vi "GateCharge_Main.vi"() -> ()   [LabVIEW 2020]
uses:
  Global 1.vi
panel:
  in  "Median Filter Rank":i32=30
  out "Cluster 4":T1
  out "CURRENT RESULT":dbl[](array[numeric])
  in  "START TEST":bool
  out "Started":bool
  out "Elapsed time (minutes)":dbl
  out "start time":timestamp
  out "Oscilloscope Capture":waveform(dbl)[](graph)
  out "ALL RESULT Array":dbl[][](array[numeric])
  out "TEST#   |  Elapsed Time (minutes)":dbl[][](array[numeric])
  out "Gate Charge :\nTotal Test Time (minutes)":dbl
  in  "Finish?":bool
  out "Cluster 3":T2
  out "Cluster 2":T3
  out "Cluster 1":T4
  in  "Cluster : Setting":T5={"[-ve] VGE (V)"=0.0, "VCE (V)"=0.0, "ICE (A)"=0.0, "TEKTRONIX"="", "PROJECT #"="", "TEMPERATURE (C)"=0.0, "RG (Ohm)"=0.0, "DUT #"=1, "REQUEST #"="", "TEST #"=1, "IGE (mA)"=0.0, "[+ve] VGE (V)"=0.0}
  out "error out":errorcluster
  in  "error in (no error)":errorcluster
  # "PRODUCED BY : AFIQAH HASBULLAH ( SBN CZ ENG : 2022)"
  # "AC MODULE : GATE CHARGE"
  # "Column 0"
  # "Column 1"
  # "Column 2"
  # "Column 3"
  # "Column 4"
  # "Column 5"
  # "Column 6"
  # "Column 7"
  # "Column 8"
  # "Column 9"
  # "Column 10"
  # "Column 11"
  # "Column 12"
  # "Qge\n(nC)"
  # "Qgc\n(nC)"
  # "Qgtot\n(nC)"
  # "Vpl\n(V)"
  # "Vce"
  # "Ice"
  # "[-ve]Vge"
  # "[+ve]Vge"
  # "Rg"
  # "Temperature"
  # "DUT  #"
  # "TEST #"
  # "Ige"
  # "< Press 2 times >"
  # "Column 0"
  # "Column 1"
  # "Column 2"
  # "Column 3"
  # "Column 4"
  # "Column 5"
  # "Column 6"
  # "Column 7"
  # "Column 8"
  # "Column 9"
  # "Column 10"
  # "Column 11"
  # "Column 12"
  # "Qge\n(nC)"
  # "Qgc\n(nC)"
  # "Qgtot\n(nC)"
  # "Vpl\n(V)"
  # "Vce"
  # "Ice"
  # "[-ve]Vge"
  # "[+ve]Vge"
  # "Rg"
  # "Temperature"
  # "DUT  #"
  # "TEST #"
  # "Ige"
  # "Done  Qgtot  &  Vpl  Acquisition"
  # "Done  Qgc  Acquisition"
  # "Done  Qge  Acquisition"
  # "Done Exporting image of Overall Waveform"
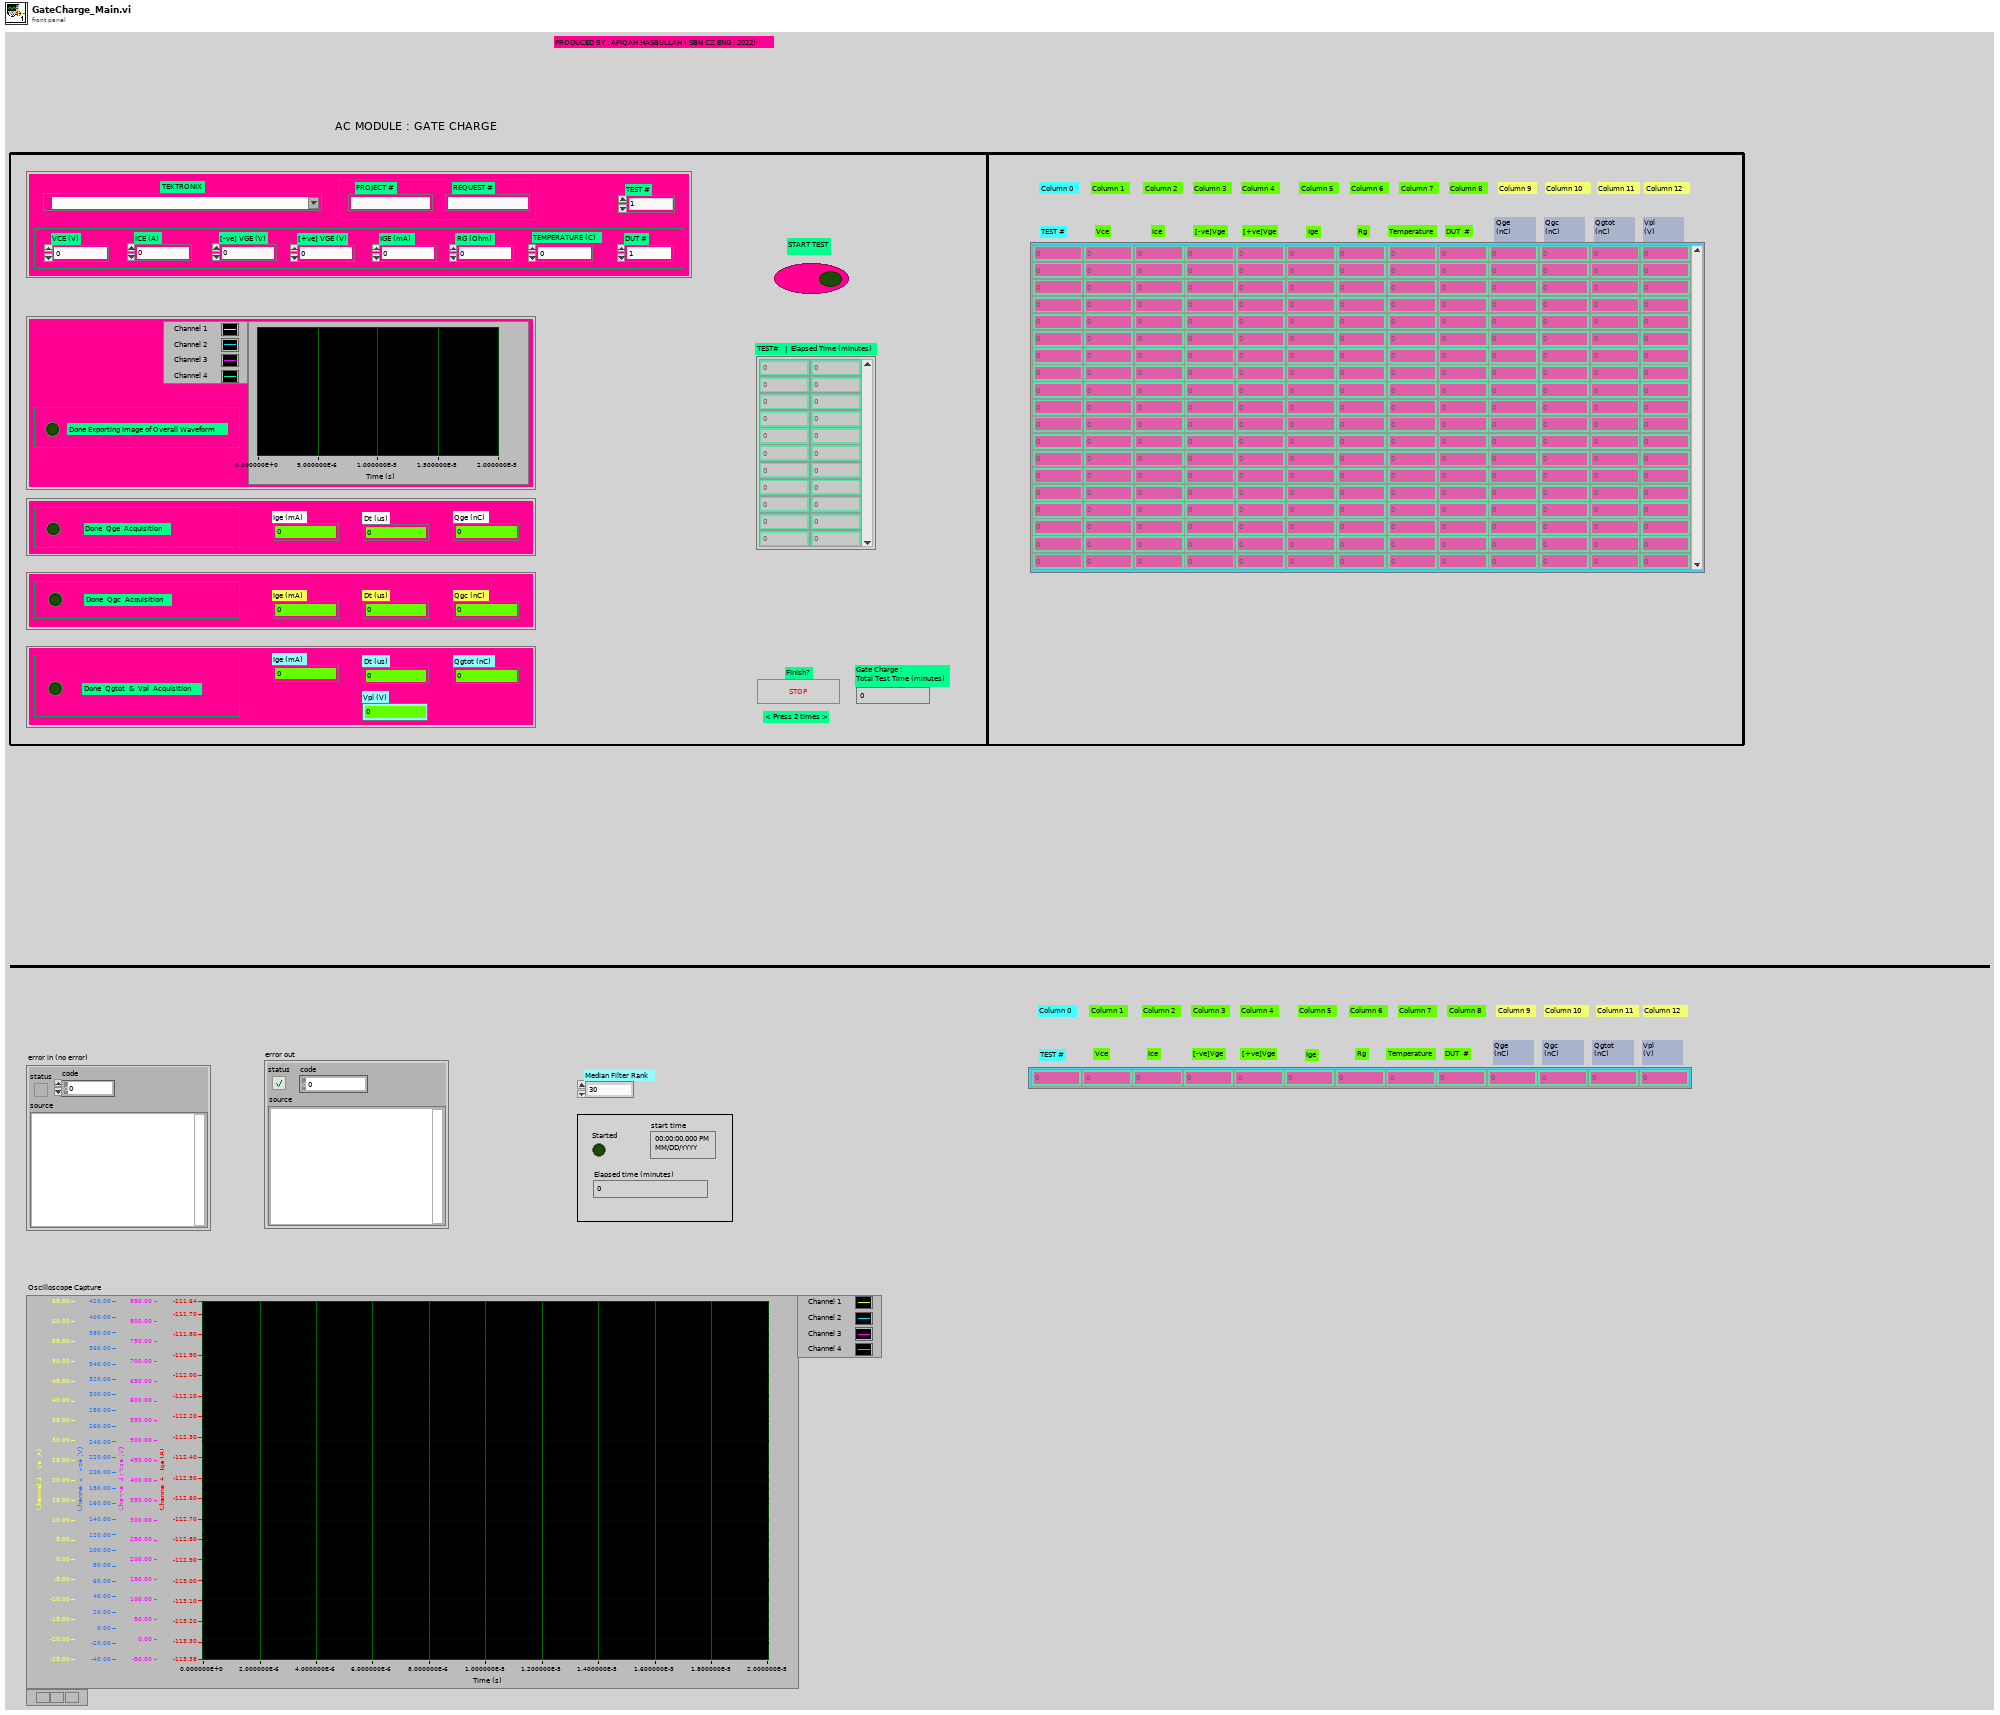
[diagram p1: front panel]
types:
  T1 = cluster{"Ige (mA)":dbl, "Qgtot (nC)":dbl, "Dt (us)":dbl, "LED 4":bool, "Vpl (V)":dbl}
  T2 = cluster{"Ige (mA)":dbl, "Dt (us)":dbl, "Qgc (nC)":dbl, "LED 3":bool}
  T3 = cluster{"Qge (nC)":dbl, "Ige (mA)":dbl, "Dt (us)":dbl, "LED 2":bool}
  T4 = cluster{"LED 1":bool, "Oscilloscope Capture":waveform(dbl)[]}
  T5 = cluster{"[-ve] VGE (V)":dbl, "VCE (V)":dbl, "ICE (A)":dbl, "TEKTRONIX":refnum<visa-resource-name>, "PROJECT #":string, "TEMPERATURE (C)":dbl, "RG (Ohm)":dbl, "DUT #":i32, "REQUEST #":string, "TEST #":i32, "IGE (mA)":dbl, "[+ve] VGE (V)":dbl}
  T6 = cluster{"Ige (mA)":dbl, "Qgtot (nC)":dbl, "Dt (us)":dbl, "LED 3":bool, "Vpl (V)":dbl}
  T7 = cluster{"Di/Dt (A/us)":dbl, "Di (A)":dbl, "Dt (ns)":dbl, "LED 2":bool}
  T8 = typedef "imagedata.ctl" = cluster{"image type":i32, "image depth":i32, "image":u8[], "mask":u8[], "colors":u32[], "Rectangle":cluster{"left":i16, "top":i16, "right":i16, "bottom":i16}}
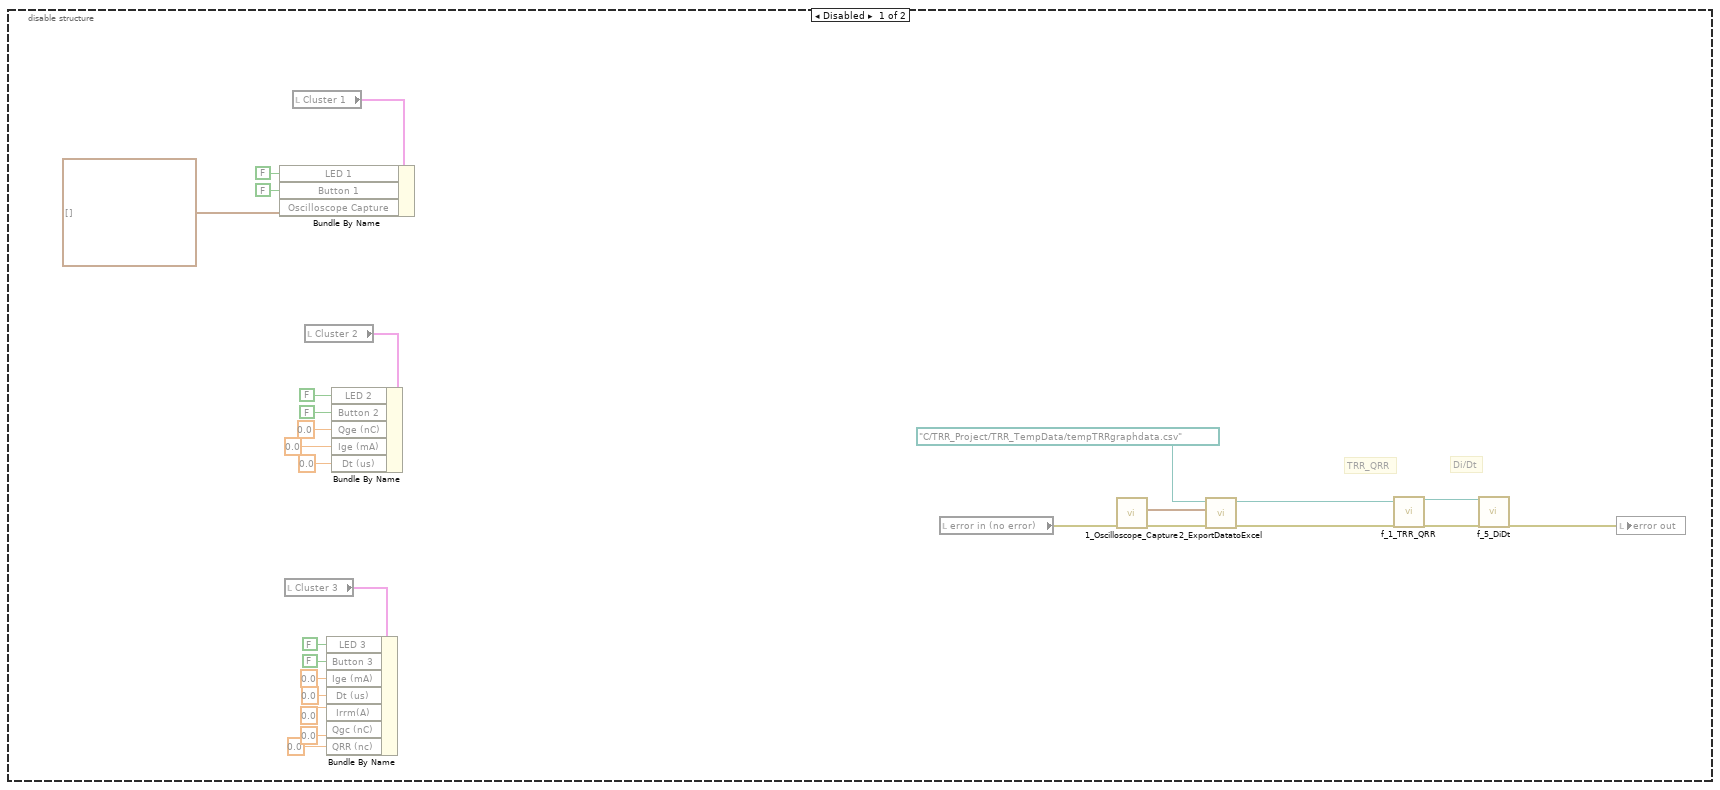
[diagram p3: hidden frame]
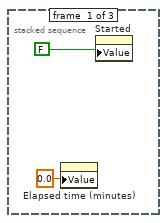
[diagram p4: hidden frame]
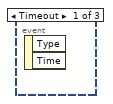
[diagram p6: hidden frame]
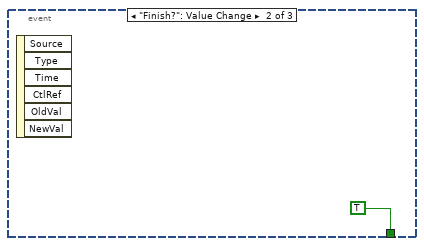
[diagram p7: hidden frame]
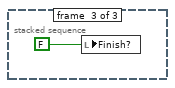
[diagram p9: hidden frame]
diagram:
  w1 = 30 ("Median Filter Rank")
  w18 = errorcluster {"status"=FALSE, "code"=0, "source"=""} ("error out")
  w5 = FALSE ("Started")
  w17 = 0.0 ("TRR :\nTotal Test Time (minutes)")
  n1 = flat-sequence {
    tunnel: [w28] -> w8
    tunnel: w8 -> [w29]
    tunnel: [w30] -> w7
    tunnel: w7 -> [w296]
    tunnel: [w291] -> w6
    tunnel: w6 -> [w322]
    frame #0 {
      # "IN"
      n2 = local read "error in (no error)"() -> (w28:errorcluster)
    }
    frame #1 {
      n3 = while {
        shift-right: [w33] -> w30
        shift-left: w29 -> [w32]
        stop <- w34 stop-if-true
        n4 = local read "START TEST"() -> (w36:bool)
        n5 = case shown="True" w36 {
          tunnel: w32 -> [w37 w57]
          tunnel: [w37 w38] -> w33
          frame False {
          }
          frame True {
            n6 = flat-sequence {
              tunnel: w57 -> [w59]
              tunnel: [w59] -> w51
              tunnel: w51 -> [w80]
              tunnel: [w80] -> w50
              tunnel: [w78] -> w49
              tunnel: [w77] -> w48
              tunnel: [w76] -> w47
              tunnel: [w75] -> w46
              tunnel: [w74] -> w45
              tunnel: [w73] -> w44
              tunnel: [w72] -> w43
              tunnel: [w70] -> w42
              tunnel: [w69] -> w41
              tunnel: w50 -> [w96]
              tunnel: [w96] -> w56
              tunnel: w49 -> [w95]
              tunnel: w48 -> [w94]
              tunnel: w47 -> [w93]
              tunnel: w46 -> [w92]
              tunnel: w45 -> [w91]
              tunnel: w44 -> [w90]
              tunnel: w43 -> [w89]
              tunnel: w42 -> [w82]
              tunnel: w41 -> [w81]
              tunnel: w56 -> [w123]
              tunnel: [w122] -> w55
              tunnel: w55 -> [w160]
              tunnel: [w156] -> w54
              tunnel: w54 -> [w198]
              tunnel: [w195] -> w40
              tunnel: w40 -> [w230]
              tunnel: [w228] -> w39
              tunnel: w39 -> [w269]
              tunnel: [w269] -> w53
              tunnel: w53 -> [w277]
              tunnel: [w277] -> w52
              tunnel: w52 -> [w286]
              tunnel: [w286] -> w38
              frame #0 {
                # "Initialize"
                n7 = local read "Median Filter Rank"() -> (w58:i32)
                n8 = Initialize Array(0.0 ("element"), 13 ("dimension size")) -> (w64:dbl[])
                n9 = local write "Cluster 4"(T6 {"Ige (mA)"=0.0, "Qgtot (nC)"=0.0, "Dt (us)"=0.0, "LED 3"=FALSE, "Vpl (V)"=0.0} ("Cluster 4")) -> ()
                n10 = local write "Cluster 3"(T2 {"Ige (mA)"=0.0, "Dt (us)"=0.0, "Qgc (nC)"=0.0, "LED 3"=FALSE} ("Cluster 3")) -> ()
                n11 = local write "Cluster 2"(T7 {"Di/Dt (A/us)"=0.0, "Di (A)"=0.0, "Dt (ns)"=0.0, "LED 2"=FALSE} ("Cluster 2")) -> ()
                n12 = local write "Oscilloscope Capture"(waveform(dbl)[] [] ("Oscilloscope Capture")) -> ()
                n13 = local write "CURRENT RESULT"(w64) -> ()
                n14 = Wait (ms)(milliseconds to wait=u32 500) -> ()  [unwired: 1 out]
                n15 = global write "Global 1.vi" "Median Filter Rank"(w58) -> ()
                n16 = local write "Cluster 1"(T4 {"LED 1"=FALSE, "Oscilloscope Capture"=[]} ("Cluster 1")) -> ()
              }
              frame #1 {
                n17 = local read "Cluster : Setting"() -> (w79:T5)
                n18 = Unbundle By Name(w79) -> ("TEST #"=w78:i32, "VCE (V)"=w77:dbl, "ICE (A)"=w76:dbl, "[-ve] VGE (V)"=w75:dbl, "[+ve] VGE (V)"=w74:dbl, "IGE (mA)"=w73:dbl, "RG (Ohm)"=w72:dbl, "TEMPERATURE (C)"=w70:dbl, "DUT #"=w69:i32)
                n19 = Wait (ms)(milliseconds to wait=u32 300) -> ()  [unwired: 1 out]
              }
              frame #2 {
                # "Column 8 = DUT#"
                # "Column 7 = Temperature"
                # "Column 6 = Rg"
                # "Column 5 = Ige"
                # "Column 4 = [+ve]Vge"
                # "Column 3 = [-ve]Vge"
                # "Column 2 = ICE"
                # "Column 1 = VCE"
                # "Column 0 = TEST#"
                # "Insert Test Condition"
                n20 = Wait (ms)(milliseconds to wait=u32 300) -> ()  [unwired: 1 out]
                n21 = local read "CURRENT RESULT"() -> (w87:dbl[])
                n22 = local read "CURRENT RESULT"() -> (w99:dbl[])
                n23 = local read "CURRENT RESULT"() -> (w101:dbl[])
                n24 = local read "CURRENT RESULT"() -> (w84:dbl[])
                n25 = local read "CURRENT RESULT"() -> (w103:dbl[])
                n26 = local read "CURRENT RESULT"() -> (w104:dbl[])
                n27 = local read "CURRENT RESULT"() -> (w111:dbl[])
                n28 = local read "CURRENT RESULT"() -> (w107:dbl[])
                n29 = local read "CURRENT RESULT"() -> (w109:dbl[])
                n30 = Replace Array Subset(array=w111, new element=w95, index=0) -> (w110:dbl[])
                n31 = Replace Array Subset(array=w109, new element=w94, index=1) -> (w108:dbl[])
                n32 = Replace Array Subset(array=w107, new element=w93, index=2) -> (w106:dbl[])
                n33 = Replace Array Subset(array=w104, new element=w92, index=3) -> (w105:dbl[])
                n34 = Replace Array Subset(array=w87, new element=w82, index=7) -> (w88:dbl[])
                n35 = Replace Array Subset(array=w99, new element=w89, index=6) -> (w98:dbl[])
                n36 = Replace Array Subset(array=w103, new element=w91, index=4) -> (w102:dbl[])
                n37 = Replace Array Subset(array=w101, new element=w90, index=5) -> (w100:dbl[])
                n38 = Replace Array Subset(array=w84, new element=w81, index=8) -> (w83:dbl[])
                n39 = local write "CURRENT RESULT"(w110) -> ()
                n40 = local write "CURRENT RESULT"(w108) -> ()
                n41 = local write "CURRENT RESULT"(w106) -> ()
                n42 = local write "CURRENT RESULT"(w105) -> ()
                n43 = local write "CURRENT RESULT"(w102) -> ()
                n44 = local write "CURRENT RESULT"(w100) -> ()
                n45 = local write "CURRENT RESULT"(w88) -> ()
                n46 = local write "CURRENT RESULT"(w98) -> ()
                n47 = local write "CURRENT RESULT"(w83) -> ()
              }
              frame #3 {
                n48 = Wait (ms)(milliseconds to wait=u32 300) -> ()  [unwired: 1 out]
                n49 = flat-sequence {
                  tunnel: w123 -> [w130]
                  tunnel: [w125] -> w120
                  tunnel: [w135] -> w119
                  tunnel: w120 -> [w134]
                  tunnel: [w151] -> w122
                  tunnel: w119 -> [w151]
                  frame #0 {
                    n50 = local read "Cluster : Setting"() -> (w129:T5)
                    n51 = Unbundle By Name(w129) -> ("TEKTRONIX"=w128:refnum<visa-resource-name>)
                    n52 = call "1_Oscilloscope_Capture.vi"("error in (no error)"=w130, "VISA Resource Name"=w128) -> ("error out"=w126:errorcluster, "Waveform Graph"=w124:waveform(dbl)[])  [unwired: 7 in, 1 out]
                    n53 = local write "Oscilloscope Capture"(w124) -> ()
                    n54 = local read "Cluster 1"() -> (w133:T4)
                    n55 = Bundle By Name(cluster=w133, "Oscilloscope Capture"=w124) -> (w132:T4)
                    n56 = local write "Cluster 1"(w132) -> ()
                    n57 = Wait (ms)(milliseconds to wait=u32 300) -> ()  [unwired: 1 out]
                    n58 = call "2_ExportDatatoExcel.vi"("error in (no error)"=w126, "Waveform Graph"=w124, "file path (IN)"=path "C:/GateCharge_Project/GateCharge_TempData/tempGateChargedata.csv") -> ("error out"=w125:errorcluster)  [unwired: 7 in, 1 out]
                  }
                  frame #1 {
                    w147 = "_"
                    n59 = local read "Cluster : Setting"() -> (w142:T5)
                    n60 = Unbundle By Name(w142) -> ("PROJECT #"=w139:string, "REQUEST #"=w138:string, "TEST #"=w141:i32)
                    n61 = invoke on="Oscilloscope Capture" class="WFGraph (strict)" method="Get Image"(error in=w134) -> (error out=w143:errorcluster, "image data"=w144:T8)  [unwired: 5 in, 4 out]
                    n62 = Format Value(format string="%d", value (0)=w141) -> (output string=w137:string)  [unwired: 1 in]
                    n63 = Concatenate Strings("C:\\GateCharge_Project\\GateCharge_Image\\" ("string"), w139, w147, w138, w147, w137, w147, "GateCharge_FullWaveform" ("string"), ".png" ("string")) -> (w150:string)
                    n64 = String To Path(string=w150) -> (path=w149:path)
                    n65 = call <vilib>:"Write PNG File.vi"("error in (no error)"=w143, "image data"=w144, "path to PNG file"=w149) -> ("error out"=w135:errorcluster)  [unwired: 7 in, 1 out]
                    n66 = Wait (ms)(milliseconds to wait=u32 300) -> ()  [unwired: 1 out]
                  }
                  frame #2 {
                    n67 = local read "Cluster 1"() -> (w155:T4)
                    n68 = Bundle By Name(cluster=w155, "LED 1"=TRUE) -> (w153:T4)
                    n69 = Wait (ms)(milliseconds to wait=u32 300) -> ()  [unwired: 1 out]
                    n70 = local write "Cluster 1"(w153) -> ()
                  }
                }
              }
              frame #4 {
                # "Step 1 : Qge"
                n71 = Wait (ms)(milliseconds to wait=u32 300) -> ()  [unwired: 1 out]
                n72 = flat-sequence {
                  tunnel: w160 -> [w163]
                  tunnel: [w163] -> w159
                  tunnel: [w164] -> w162
                  tunnel: w159 -> [w168]
                  tunnel: [w167] -> w157
                  tunnel: w162 -> [w183]
                  tunnel: [w181] -> w158
                  tunnel: w157 -> [w181]
                  tunnel: w158 -> [w187]
                  tunnel: [w187] -> w156
                  frame #0 {
                  }
                  frame #1 {
                    # "Qge"
                    n73 = local read "Cluster : Setting"() -> (w179:T5)
                    n74 = Unbundle By Name(w179) -> ("[+ve] VGE (V)"=w173:dbl, "[-ve] VGE (V)"=w174:dbl, "PROJECT #"=w171:string, "REQUEST #"=w170:string, "TEST #"=w180:i32, "IGE (mA)"=w166:dbl)
                    n75 = Format Value(format string="%d", value (0)=w180) -> (output string=w169:string)  [unwired: 1 in]
                    n76 = call "f_1_Qge.vi"("file path (IN)"=path "C:/GateCharge_Project/GateCharge_TempData/tempGateChargedata.csv", "Project #"=w171, "Request #"=w170, "TEST #"=w169, "error in (no error)"=w168, "VGE (-ve)"=w174, "VGE (+ve)"=w173) -> ("Qge - Delta Time (us)"=w165:dbl, "error out"=w167:errorcluster)  [unwired: 5 in, 6 out]
                    n77 = Multiply(x=w166, y=w165) -> (x*y=w164:dbl)
                    n78 = local read "Cluster 2"() -> (w177:T3)
                    n79 = Bundle By Name(cluster=w177, "Ige (mA)"=w166, "Dt (us)"=w165, "Qge (nC)"=w164) -> (w176:T3)
                    n80 = Wait (ms)(milliseconds to wait=u32 300) -> ()  [unwired: 1 out]
                    n81 = local write "Cluster 2"(w176) -> ()
                  }
                  frame #2 {
                    # "Column 9 = Qge"
                    n82 = local read "CURRENT RESULT"() -> (w185:dbl[])
                    n83 = Wait (ms)(milliseconds to wait=u32 300) -> ()  [unwired: 1 out]
                    n84 = Replace Array Subset(array=w185, new element=w183, index=9) -> (w184:dbl[])
                    n85 = local write "CURRENT RESULT"(w184) -> ()
                  }
                  frame #3 {
                    n86 = local read "Cluster 2"() -> (w190:T3)
                    n87 = Bundle By Name(cluster=w190, "LED 2"=TRUE ("LED 1")) -> (w191:T3)
                    n88 = Wait (ms)(milliseconds to wait=u32 300) -> ()  [unwired: 1 out]
                    n89 = local write "Cluster 2"(w191) -> ()
                  }
                }
              }
              frame #5 {
                # "Step 2 : Qgc"
                n90 = Wait (ms)(milliseconds to wait=u32 300) -> ()  [unwired: 1 out]
                n91 = flat-sequence {
                  tunnel: w198 -> [w199]
                  tunnel: [w199] -> w197
                  tunnel: w197 -> [w203]
                  tunnel: [w201] -> w193
                  tunnel: [w200] -> w192
                  tunnel: [w217] -> w196
                  tunnel: w193 -> [w218]
                  tunnel: w192 -> [w217]
                  tunnel: w196 -> [w223]
                  tunnel: [w223] -> w195
                  frame #0 {
                  }
                  frame #1 {
                    # "Qgc"
                    n92 = local read "Cluster : Setting"() -> (w211:T5)
                    n93 = Unbundle By Name(w211) -> ("[+ve] VGE (V)"=w208:dbl, "[-ve] VGE (V)"=w209:dbl, "PROJECT #"=w206:string, "REQUEST #"=w205:string, "TEST #"=w210:i32, "IGE (mA)"=w215:dbl)
                    n94 = Format Value(format string="%d", value (0)=w210) -> (output string=w204:string)  [unwired: 1 in]
                    n95 = call "f_2_Qgc.vi"("file path (IN)"=path "C:/GateCharge_Project/GateCharge_TempData/tempGateChargedata.csv", "Project #"=w206, "Request #"=w205, "TEST #"=w204, "error in (no error)"=w203, "VGE (-ve)"=w209, "VGE (+ve)"=w208) -> ("Qgc - Delta Time (us)"=w202:dbl, "error out"=w200:errorcluster)  [unwired: 5 in, 6 out]
                    n96 = Multiply(x=w215, y=w202) -> (x*y=w201:dbl)
                    n97 = local read "Cluster 3"() -> (w213:T2)
                    n98 = Bundle By Name(cluster=w213, "Ige (mA)"=w215, "Dt (us)"=w202, "Qgc (nC)"=w201) -> (w214:T2)
                    n99 = local write "Cluster 3"(w214) -> ()
                    n100 = Wait (ms)(milliseconds to wait=u32 300) -> ()  [unwired: 1 out]
                  }
                  frame #2 {
                    # "Column 10 = Qgc"
                    n101 = local read "CURRENT RESULT"() -> (w221:dbl[])
                    n102 = Wait (ms)(milliseconds to wait=u32 300) -> ()  [unwired: 1 out]
                    n103 = Replace Array Subset(array=w221, new element=w218, index=10) -> (w220:dbl[])
                    n104 = local write "CURRENT RESULT"(w220) -> ()
                  }
                  frame #3 {
                    n105 = local read "Cluster 3"() -> (w226:T2)
                    n106 = Bundle By Name(cluster=w226, "LED 3"=TRUE ("LED 1")) -> (w227:T2)
                    n107 = Wait (ms)(milliseconds to wait=u32 300) -> ()  [unwired: 1 out]
                    n108 = local write "Cluster 3"(w227) -> ()
                  }
                }
              }
              frame #6 {
                # "Step 3 : Qgtot & Vpl"
                n109 = flat-sequence {
                  tunnel: w230 -> [w235]
                  tunnel: [w235] -> w234
                  tunnel: w234 -> [w245]
                  tunnel: [w246] -> w233
                  tunnel: [w244] -> w232
                  tunnel: [w236] -> w229
                  tunnel: [w258] -> w231
                  tunnel: w233 -> [w259]
                  tunnel: w232 -> [w258]
                  tunnel: w229 -> [w254]
                  tunnel: w231 -> [w264]
                  tunnel: [w264] -> w228
                  frame #0 {
                  }
                  frame #1 {
                    # "Qgtot & Vpl"
                    n110 = local read "Cluster : Setting"() -> (w248:T5)
                    n111 = Unbundle By Name(w248) -> ("[+ve] VGE (V)"=w242:dbl, "[-ve] VGE (V)"=w243:dbl, "PROJECT #"=w240:string, "REQUEST #"=w239:string, "TEST #"=w247:i32, "IGE (mA)"=w252:dbl)
                    n112 = Format Value(format string="%d", value (0)=w247) -> (output string=w238:string)  [unwired: 1 in]
                    n113 = call "f_3_Qgtot_Vpl.vi"("file path (IN)"=path "C:/GateCharge_Project/GateCharge_TempData/tempGateChargedata.csv", "Project #"=w240, "Request #"=w239, "TEST #"=w238, "error in (no error)"=w245, "VGE (-ve)"=w243, "VGE (+ve)"=w242) -> ("Vpl"=w236:dbl, "Qgtot - Delta Time (us)"=w237:dbl, "error out"=w244:errorcluster)  [unwired: 4 in, 6 out]
                    n114 = Multiply(x=w252, y=w237) -> (x*y=w246:dbl)
                    n115 = local read "Cluster 4"() -> (w250:T1)
                    n116 = Bundle By Name(cluster=w250, "Ige (mA)"=w252, "Dt (us)"=w237, "Qgtot (nC)"=w246, "Vpl (V)"=w236) -> (w251:T1)
                    n117 = local write "Cluster 4"(w251) -> ()
                    n118 = Wait (ms)(milliseconds to wait=u32 300) -> ()  [unwired: 1 out]
                  }
                  frame #2 {
                    # "Column 12 = Vpl"
                    # "Column 11 = Qgtot"
                    n119 = local read "CURRENT RESULT"() -> (w262:dbl[])
                    n120 = local read "CURRENT RESULT"() -> (w256:dbl[])
                    n121 = Wait (ms)(milliseconds to wait=u32 300) -> ()  [unwired: 1 out]
                    n122 = Replace Array Subset(array=w262, new element=w259, index=11) -> (w261:dbl[])
                    n123 = Replace Array Subset(array=w256, new element=w254, index=12) -> (w257:dbl[])
                    n124 = local write "CURRENT RESULT"(w261) -> ()
                    n125 = local write "CURRENT RESULT"(w257) -> ()
                  }
                  frame #3 {
                    n126 = local read "Cluster 4"() -> (w267:T1)
                    n127 = Bundle By Name(cluster=w267, "LED 4"=TRUE ("LED 1")) -> (w268:T1)
                    n128 = Wait (ms)(milliseconds to wait=u32 300) -> ()  [unwired: 1 out]
                    n129 = local write "Cluster 4"(w268) -> ()
                  }
                }
              }
              frame #7 {
                # "Update Data in All Result Array"
                n130 = local read "Cluster : Setting"() -> (w276:T5)
                n131 = Unbundle By Name(w276) -> ("TEST #"=w274:i32)
                n132 = local read "CURRENT RESULT"() -> (w272:dbl[])
                n133 = local read "ALL RESULT Array"() -> (w273:dbl[][])
                n134 = Wait (ms)(milliseconds to wait=u32 300) -> ()  [unwired: 1 out]
                n135 = Decrement(x=w274) -> (x-1=w275:i32)
                n136 = Replace Array Subset(array=w273, new element=w272, index (row)=w275) -> (w271:dbl[][])  [unwired: 1 in]
                n137 = local write "ALL RESULT Array"(w271) -> ()
              }
              frame #8 {
                # "Increment TEST# & DUT#"
                n138 = local read "Cluster : Setting"() -> (w285:T5)
                n139 = Unbundle By Name(w285) -> ("TEST #"=w284:i32, "DUT #"=w283:i32)
                n140 = Increment(x=w284) -> (x+1=w280:i32)
                n141 = Increment(x=w283) -> (x+1=w279:i32)
                n142 = local read "Cluster : Setting"() -> (w282:T5)
                n143 = Wait (ms)(milliseconds to wait=u32 200) -> ()  [unwired: 1 out]
                n144 = Bundle By Name(cluster=w282, "TEST #"=w280, "DUT #"=w279) -> (w281:T5)
                n145 = local write "Cluster : Setting"(w281) -> ()
              }
              frame #9 {
                n146 = local write "START TEST"(FALSE ("START TEST")) -> ()
                n147 = local write "Started"(FALSE ("Started")) -> ()
                n148 = Wait (ms)(milliseconds to wait=u32 1000) -> ()  [unwired: 1 out]
              }
            }
          }
        }
        n149 = Wait (ms)(milliseconds to wait=u32 300) -> ()  [unwired: 1 out]
        n150 = local read "Finish?"() -> (w34:bool)
      }
      n151 = Wait (ms)(milliseconds to wait=u32 300) -> ()  [unwired: 1 out]
    }
    frame #2 {
      # "Minutes"
      # "Export to Excel"
      n152 = local read "Cluster : Setting"() -> (w305:T5)
      n153 = local read "TEST#   |  Elapsed Time (minutes)"() -> (w301:dbl[][])
      n154 = Unbundle By Name(w305) -> ("TEST #"=w302:i32)
      n155 = Index Array(array=w301, index (col)=1 ("disabled index (col)")) -> (element=w304:dbl[])  [unwired: 1 in]
      n156 = local read "ALL RESULT Array"() -> (w306:dbl[][])
      n157 = Decrement(x=w302) -> (x-1=w303:i32)
      n158 = Split 1D Array(array=w304, index=w303) -> (first subarray=w298:dbl[])  [unwired: 1 out]
      n159 = Decrement(x=w302) -> (x-1=w307:i32)
      n160 = local read "Cluster : Setting"() -> (w313:T5)
      n161 = for {
        tunnel: w298 -> [w321] mode=indexing
        shift-right: [w318] -> w297
        shift-left: 0.0 -> [w320]
        shift-right: [w319] -> w294
        shift-left: w296 -> [w319]
        n162 = Add(x=w321, y=w320) -> (x+y=w318:dbl)
        n163 = local write "Gate Charge :\nTotal Test Time (minutes)"(w318) -> ()
      }
      n164 = Array Subset(array=w306, index (row)=0 ("index"), length (row)=w307, index (col)=0 ("index"), length (col)=13 ("length")) -> (w292:dbl[][])
      n165 = Unbundle By Name(w313) -> ("PROJECT #"=w312:string, "REQUEST #"=w311:string)
      n166 = call "O_Data_to_Excel.vi"("error in (no error)"=w296, "ALL RESULT Array"=w292, "REQUEST #"=w311, "PROJECT #"=w312) -> ("error out"=w293:errorcluster)  [unwired: 7 in]
      n167 = Wait (ms)(milliseconds to wait=u32 400) -> ()  [unwired: 1 out]
      n168 = local write "Gate Charge :\nTotal Test Time (minutes)"(w297) -> ()
      n169 = Merge Errors(w293, w294) -> (w295:errorcluster)
      n170 = while {
        shift-right: [w314] -> w291
        shift-left: w295 -> [w315]
        stop <- w316 stop-if-true
        n171 = call "Display Message to User"("error in (no error)"=w315) -> ("error out"=w314:errorcluster, "OK"=w316:bool)  [unwired: 9 in]
        n172 = Wait (ms)(milliseconds to wait=u32 100) -> ()  [unwired: 1 out]
      }
    }
    frame #3 {
      # "OUT"
      n173 = local write "error out"(w322) -> ()
    }
  }
  n174 = local read "Cluster : Setting"() -> (w16:T5)
  n175 = Bundle By Name(cluster=w16, "TEST #"=1, "DUT #"=1) -> (w15:T5)
  n176 = local write "Cluster : Setting"(w15) -> ()
  n177 = Initialize Array(0.0 ("element"), 100 ("dimension size"), 2 ("dimension size")) -> (→"TEST#   |  Elapsed Time (minutes)":dbl[][])
  n178 = Initialize Array(0.0 ("element"), 100 ("dimension size"), 13 ("dimension size")) -> (→"ALL RESULT Array":dbl[][])
  n179 = Initialize Array(0.0 ("element"), 13 ("dimension size")) -> (→"CURRENT RESULT":dbl[])
  n180 = local write "START TEST"(w5) -> ()
  n181 = local write "Started"(w5) -> ()
  n182 = local write "Finish?"(w5) -> ()
  n183 = local write "error out"(w18) -> ()
  n184 = local write "error in (no error)"(w18) -> ()
  n185 = global write "Global 1.vi" "Median Filter Rank"(w1) -> ()
  n186 = local write "Median Filter Rank"(w1) -> ()
  n187 = disable-structure shown="Enabled" {
    frame Disabled {
      # "Di/Dt"
      # "TRR_QRR"
      n188 = local read "Cluster 3"() -> (w339:T2)
      n189 = local read "Cluster 1"() -> (w349:T4)
      n190 = Bundle By Name(cluster=w349, "LED 1"=FALSE, "Button 1"=FALSE, "Oscilloscope Capture"=waveform(dbl)[] []) -> ()  [unwired: 1 out]
      n191 = local read "Cluster 2"() -> (w348:T3)
      n192 = Bundle By Name(cluster=w339, "LED 3"=FALSE, "Button 3"=FALSE, "Ige (mA)"=0.0 ("Ta (ns)"), "Dt (us)"=0.0 ("Tb (ns)"), "Irrm(A)"=0.0, "Qgc (nC)"=0.0 ("TRR (ns)"), "QRR (nc)"=0.0) -> ()  [unwired: 1 out]
      n193 = Bundle By Name(cluster=w348, "LED 2"=FALSE, "Button 2"=FALSE, "Qge (nC)"=0.0 ("Di/Dt (A/us)"), "Ige (mA)"=0.0 ("Di (A)"), "Dt (us)"=0.0 ("Dt (ns)")) -> ()  [unwired: 1 out]
      n194 = local read "error in (no error)"() -> (w330:errorcluster)
      n195 = call "1_Oscilloscope_Capture.vi"("error in (no error)"=w330) -> ("error out"=w324:errorcluster, "Waveform Graph"=w327:waveform(dbl)[])  [unwired: 8 in, 1 out]
      n196 = call "2_ExportDatatoExcel.vi"("error in (no error)"=w324, "Waveform Graph"=w327, "file path (IN)"=path "C:/TRR_Project/TRR_TempData/tempTRRgraphdata.csv") -> ("error out"=w326:errorcluster, "file path (OUT)"=w325:path)  [unwired: 7 in]
      n197 = call "f_1_TRR_QRR.vi"("file path (IN)"=w325, "error in (no error)"=w326) -> ("file path (OUT)"=w329:path, "error out"=w328:errorcluster)  [unwired: 9 in, 7 out]
      n198 = call "f_5_DiDt.vi"("file path (IN)"=w329, "error in (no error)"=w328) -> ("error out"=w331:errorcluster)  [unwired: 10 in, 7 out]
      n199 = local write "error out"(w331) -> ()
    }
    frame Enabled {
    }
  }
  n200 = while {
    stop <- w351 stop-if-true
    # "COPY from NI Forum :)"
    n201 = stacked-sequence {
      tunnel: [_ w354 _] -> w351
      frame #0 {
        n202 = property on="Elapsed time (minutes)" class="DigNum (strict)"("Value"=0.0 ("Elapsed time (seconds)")) -> ()  [unwired: 2 in, 2 out]
        n203 = property on="Started" class="Bool (strict)"("Value"=FALSE ("Started")) -> ()  [unwired: 2 in, 2 out]
      }
      frame #1 {
        n204 = while {
          tunnel: [w355] -> w354
          stop <- w355 stop-if-true
          n205 = local read "Started"() -> (w356:bool)
          n206 = case shown="True" w356 {
            frame False {
              # "do nothing"
            }
            frame True {
              n207 = local read "start time"() -> (w368:timestamp)
              n208 = local read "Cluster : Setting"() -> (w364:T5)
              n209 = Get Date/Time In Seconds() -> (seconds since 1Jan1904=w367:timestamp)
              n210 = Subtract(x=w367, y=w368) -> (x-y=w366:dbl)
              n211 = Divide(x=w366, y=60.0) -> (x/y=w358:dbl)
              n212 = Unbundle By Name(w364) -> ("TEST #"=w360:i32)
              n213 = local write "Elapsed time (minutes)"(w358) -> ()
              n214 = Build Array(w360, w358) -> (w361:dbl[])
              n215 = local read "TEST#   |  Elapsed Time (minutes)"() -> (w363:dbl[][])
              n216 = Decrement(x=w360) -> (x-1=w359:i32)
              n217 = Replace Array Subset(array=w363, new element=w361, index (row)=w359) -> (w362:dbl[][])  [unwired: 1 in]
              n218 = local write "TEST#   |  Elapsed Time (minutes)"(w362) -> ()
            }
          }
          n219 = local read "Finish?"() -> (w355:bool)
          n220 = Wait (ms)(milliseconds to wait=u32 10) -> ()  [unwired: 1 out]
        }
        n221 = while {
          stop <- w369 stop-if-true
          n222 = event shown="[2] \"START TEST\": Value Change" {
            selector: _ -> [_ _ _]
            dyn-events: _ -> [_ _ _]
            timeout: _ -> [_ _ _]
            tunnel: [_ TRUE FALSE] -> w369
            event Timeout {
              n223 = event-data() -> ()  [unwired: 1 in, 2 out]
            }
            event "Finish?": Value Change {
              n224 = event-data() -> ()  [unwired: 1 in, 6 out]
            }
            event "START TEST": Value Change {
              n225 = event-data() -> ()  [unwired: 1 in, 6 out]
              n226 = local read "Started"() -> (w373:bool)
              n227 = Not(x=w373) -> (.not. x?=w371:bool)
              n228 = case shown="True" w371 {
                frame False {
                }
                frame True {
                  n229 = Get Date/Time In Seconds() -> (seconds since 1Jan1904=→"start time":timestamp)
                }
              }
              n230 = local write "Started"(w371) -> ()
            }
          }
        }
      }
      frame #2 {
        n231 = local write "Finish?"(FALSE ("stop")) -> ()
      }
    }
    n232 = Wait (ms)(milliseconds to wait=u32 100) -> ()  [unwired: 1 out]
  }
  "Cluster 1" <- T4 {"LED 1"=FALSE, "Oscilloscope Capture"=[]} ("Cluster 1")
  "Cluster 2" <- T7 {"Di/Dt (A/us)"=0.0, "Di (A)"=0.0, "Dt (ns)"=0.0, "LED 2"=FALSE} ("Cluster 2")
  "Cluster 3" <- T2 {"Ige (mA)"=0.0, "Dt (us)"=0.0, "Qgc (nC)"=0.0, "LED 3"=FALSE} ("Cluster 3")
  "Gate Charge :\nTotal Test Time (minutes)" <- w17
  "Oscilloscope Capture" <- waveform(dbl)[] [] ("Oscilloscope Capture")
  "Elapsed time (minutes)" <- w17
  "Cluster 4" <- T6 {"Ige (mA)"=0.0, "Qgtot (nC)"=0.0, "Dt (us)"=0.0, "LED 3"=FALSE, "Vpl (V)"=0.0} ("Cluster 4")
